vi "Word_Write.vi"(6 "String to Write":string="A1", 8 "error in (no error)":errorcluster, 9 "Documents Rerefence In":refnum<k7>) -> (0 "error out":errorcluster)   [LabVIEW 2014]
doc: "This VI demonstrates the use of ActiveX to write a table into a Microsoft Excel worksheet."
panel:
  out "Documents Refnum Out":refnum<k7>
  in  "Word Application Reference In":refnum<k7>
  out "Word Application Reference Out":refnum<k7>
  in  "Bookmark String":string
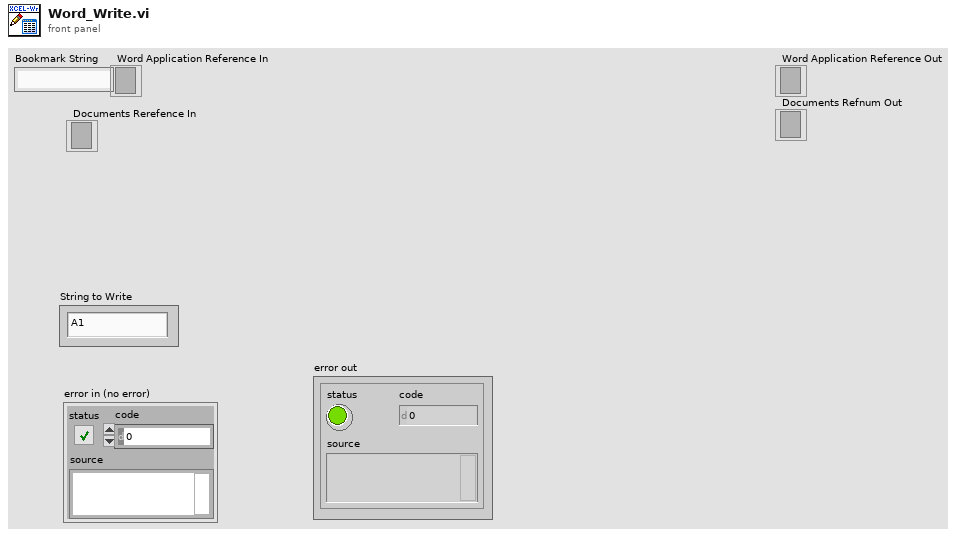
[diagram p1: front panel]
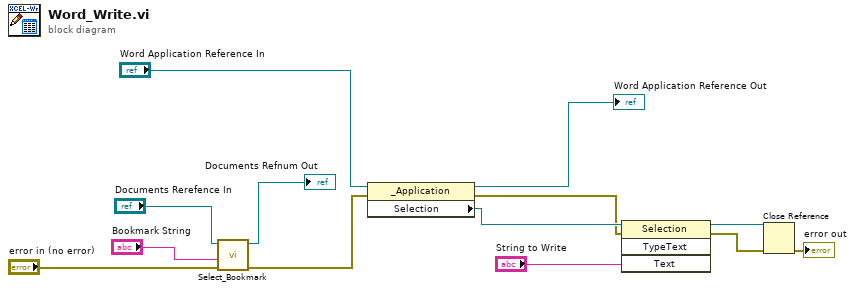
[diagram p0: block diagram]
diagram:
  n1 = call "Select_Bookmark.vi"("error in (no error)"="error in (no error)", "Bookmark String"="Bookmark String", "Documents Refnum in"="Documents Rerefence In") -> ("error out"=w7:errorcluster, "Documents Refnum Out"=→"Documents Refnum Out":refnum<k7>)  [unwired: 7 in]
  n2 = property class="_Application"(reference="Word Application Reference In", error in=w7) -> (reference out=→"Word Application Reference Out":refnum<k7>, error out=w5:errorcluster, "Selection"=w8:refnum<k7>)
  n3 = invoke class="Selection" method="TypeText"(reference=w8, error in=w5, "Text"="String to Write") -> (reference out=w2:refnum<k7>, error out=w1:errorcluster)  [unwired: 1 in, 2 out]
  n4 = Close Reference(reference=w2, error in (no error)=w1) -> (error out=→"error out":errorcluster)
